vi "To XML.vi"(8 "error in (no error)":errorcluster, 9 "Parent":refnum<k20>, 10 "Document":refnum<k20>, 11 "Coverage in":refnum<class "Coverage.lvclass">) -> (0 "error out":errorcluster)   [LabVIEW 2017, in "Cobertura.lvlib" / "Coverage.lvclass"]
uses:
  Coverage.lvclass
  Coverage.lvclass/Coverage.ctl
  <vilib>/xml/Close Reference(Node).vi
  Package/Package.lvclass
  <resource>/objmgr/DOMUserDefRef.rc
  <vilib>/xml/NI_XML.lvlib
  Cobertura.lvlib
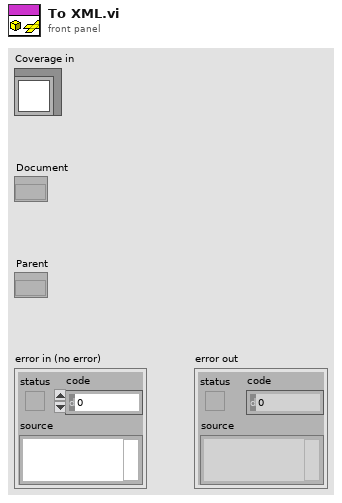
[diagram p1: front panel]
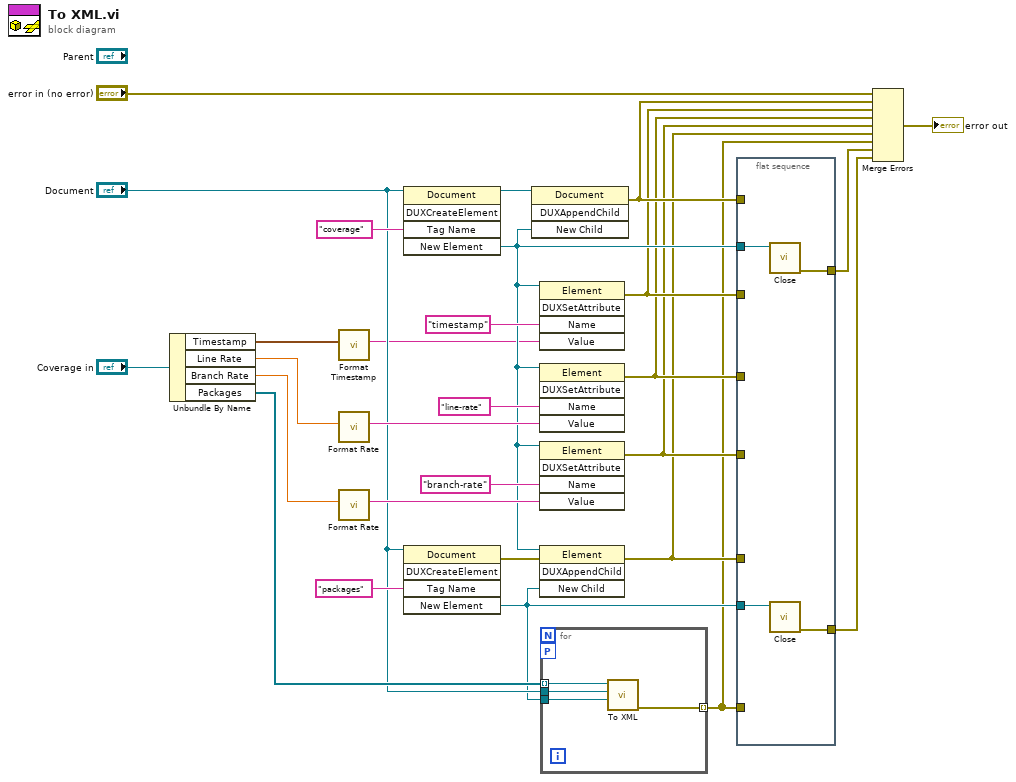
[diagram p0: block diagram]
diagram:
  n1 = Unbundle By Name("Coverage in") -> ("Timestamp"=w2:timestamp, "Line Rate"=w3:dbl, "Branch Rate"=w4:dbl, "Packages"=w22:refnum<class "Package.lvclass">[])
  n2 = call "Format Timestamp.vi"("Time Stamp"=w2) -> ("String"=w1:string)  [unwired: 10 in]
  n3 = call "Format Rate.vi"("Rate"=w3) -> ("String"=w26:string)  [unwired: 10 in]
  n4 = call "Format Rate.vi"("Rate"=w4) -> ("String"=w24:string)  [unwired: 10 in]
  n5 = invoke class="Document" method="DUXCreateElement"(reference="Document", "Tag Name"="coverage") -> (reference out=w20:refnum<k20>, "New Element"=w16:refnum<k20>)  [unwired: 3 in, 3 out]
  n6 = invoke class="Document" method="DUXCreateElement"(reference="Document", "Tag Name"="packages") -> (error out=w17:errorcluster, "New Element"=w15:refnum<k20>)  [unwired: 3 in, 3 out]
  n7 = invoke class="Document" method="DUXAppendChild"(reference=w20, "New Child"=w16) -> (error out=w14:errorcluster)  [unwired: 2 in, 3 out]
  n8 = invoke class="Element" method="DUXSetAttribute"(reference=w16, "Name"="timestamp", "Value"=w1) -> (error out=w13:errorcluster)  [unwired: 2 in, 4 out]
  n9 = invoke class="Element" method="DUXSetAttribute"(reference=w16, "Name"="line-rate", "Value"=w26) -> (error out=w12:errorcluster)  [unwired: 2 in, 4 out]
  n10 = invoke class="Element" method="DUXSetAttribute"(reference=w16, "Name"="branch-rate", "Value"=w24) -> (error out=w11:errorcluster)  [unwired: 2 in, 4 out]
  n11 = invoke class="Element" method="DUXAppendChild"(reference=w16, error in=w17, "New Child"=w15) -> (error out=w10:errorcluster)  [unwired: 1 in, 3 out]
  n12 = for {
    tunnel: w22 -> [w32] mode=indexing
    tunnel: "Document" -> [w31]
    tunnel: w15 -> [w30]
    workers-P: _ -> [_]
    tunnel: [w29] -> w9 mode=indexing
    n13 = call-dynamic "To XML.vi"("Parent"=w30, "Document"=w31, "Package in"=w32) -> ("error out"=w29:errorcluster)  [unwired: 8 in]
  }
  n14 = flat-sequence {
    tunnel: w16 -> [w36]
    tunnel: w15 -> [w35]
    tunnel: w9 -> [_]
    tunnel: w10 -> [_]
    tunnel: w11 -> [_]
    tunnel: w12 -> [_]
    tunnel: w13 -> [_]
    tunnel: w14 -> [_]
    tunnel: [w34] -> w8
    tunnel: [w33] -> w7
    frame #0 {
      n15 = call-poly <vilib>:"Close.vi"("node"=w36) -> ("error out"=w34:errorcluster)  [unwired: 8 in]
      n16 = call-poly <vilib>:"Close.vi"("node"=w35) -> ("error out"=w33:errorcluster)  [unwired: 8 in]
    }
  }
  n17 = Merge Errors("error in (no error)", w14, w13, w12, w11, w10, w9, w8, w7) -> (→"error out":errorcluster)
